vi "DAQ_6212_Trig.vi"(1 "error in":errorcluster, 2 "device name":tag="Dev1", 3 "timeout (s)":dbl=10.0, 4 "data":bool[](array[boolean])=[FALSE, FALSE, FALSE, FALSE, FALSE, FALSE, FALSE, FALSE]) -> (0 "errorout":errorcluster={"status"=TRUE, "code"=0, "source"=""})   [LabVIEW 2012]
panel:
  # "NI DAQ TTL write"
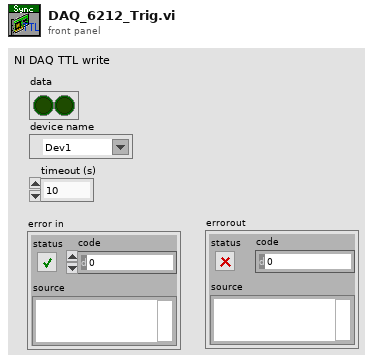
[diagram p1: front panel]
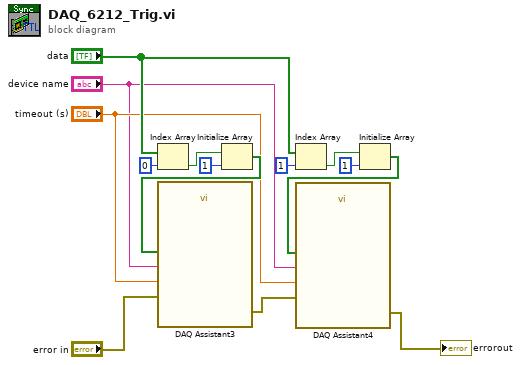
[diagram p0: block diagram]
diagram:
  n1 = Index Array(array="data", index=0) -> (element=w9:bool)
  n2 = Initialize Array(w9, 1 ("dimension size")) -> (w8:bool[])
  n3 = call "DAQ Assistant3"("data"=w8, "timeout (s)"="timeout (s)", "error in"="error in", "device name"="device name") -> ("error out"=w7:errorcluster)  [unwired: 14 in, 1 out]
  n4 = Index Array(array="data", index=1) -> (element=w3:bool)
  n5 = Initialize Array(w3, 1 ("dimension size")) -> (w1:bool[])
  n6 = call "DAQ Assistant4"("data"=w1, "timeout (s)"="timeout (s)", "error in"=w7, "device name"="device name") -> ("error out"=→"errorout":errorcluster)  [unwired: 14 in, 1 out]
